vi "Build Block Cluster.vi"(11 "UDPHandles in":u32[](array[numeric])) -> (2 "size(s)":i32, 3 "UDPBlockReadInPorts":T1[](array[typedef]) {"UDP Handle Out" format="%.0x"; "UDP Handle" format="%.0x"})   [LabVIEW 2020, in "AIM ARINC 664 Engine.lvlib" / "Implementation.lvlib" / "Rx UDP Execution Unit.lvclass"]
uses:
  Rx UDP Execution Unit.lvclass
  <instrlib>/AIM GmbH/_AIM 664/bsp/Controls/ReceiveUDPBlockRead.ctl
  <instrlib>/AIM GmbH/_AIM 664/AIM664LV.lvlib
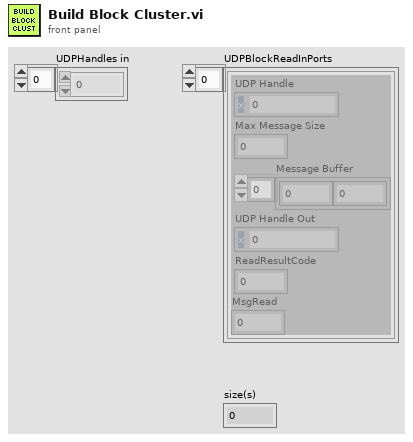
[diagram p1: front panel]
types:
  T1 = typedef "AIM664LV.lvlib/ReceiveUDPBlockRead.ctl" = cluster{"UDP Handle":u32, "Max Message Size":u32, "Message Buffer":u8[], "UDP Handle Out":u32, "ReadResultCode":i32, "MsgRead":u32}
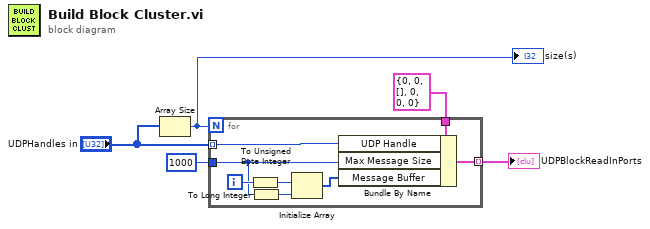
[diagram p0: block diagram]
diagram:
  n1 = Array Size(array="UDPHandles in") -> (size(s)=w4:i32)
  "size(s)" <- w4
  n2 = for {
    N: w4 -> [_]
    tunnel: "UDPHandles in" -> [w9] mode=indexing
    tunnel: [w13] -> w2 mode=indexing
    tunnel: T1 {"UDP Handle"=0, "Max Message Size"=0, "Message Buffer"=[], "UDP Handle Out"=0, "ReadResultCode"=0, "MsgRead"=0} ("UdpBlockReadInPort") -> [w7]
    tunnel: u32 1000 ("Block Size") -> [w6]
    i -> [w8]
    n3 = To Unsigned Byte Integer(number=w8) -> (unsigned 8bit integer=w12:u8)
    n4 = To Long Integer(number=w6) -> (32bit integer=w10:i32)
    n5 = Initialize Array(w12, w10) -> (w11:u8[])
    n6 = Bundle By Name(cluster=w7, "UDP Handle"=w9, "Max Message Size"=w6, "Message Buffer"=w11) -> (w13:T1)
  }
  "UDPBlockReadInPorts" <- w2
